vi "Output on.vi"(8 "error in (no error)":errorcluster, 10 "Output On":bool, 11 "E3610x in":refnum<class "E3610x.lvclass">) -> (0 "error out":errorcluster, 3 "E3610x out":refnum<class "E3610x.lvclass">)   [LabVIEW 2020, in "E3610x.lvclass"]
uses:
  E3610x.lvclass
  Instrument.lvclass
  C:/Sandbox/RF Bench/Source Code/WiSpry Test Framework/Instruments/Power Supply/Power Supply.lvclass
  C:/Sandbox/RF Bench/Source Code/WiSpry Test Framework/Instruments/Instrument.lvclass
  C:/Sandbox/RF Bench/Source Code/WiSpry Test Framework/Instruments/Power Supply/Keysight E3610x/E3610x.lvclass
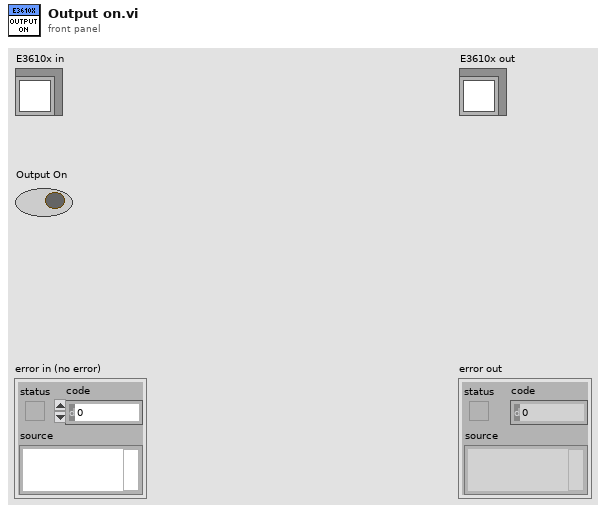
[diagram p1: front panel]
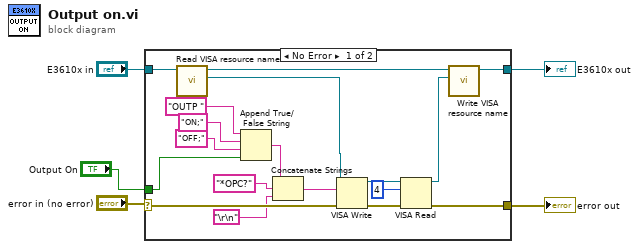
[diagram p0: block diagram]
diagram:
  n1 = case shown="No Error" "error in (no error)" {
    selector: "error in (no error)" -> [w23 w25]
    tunnel: "E3610x in" -> [w22 w24]
    tunnel: "Output On" -> [w20 _]
    tunnel: [w8 w24] -> w2
    tunnel: [w7 w25] -> w1
    frame No Error {
      n2 = call "Read VISA resource name.vi"("Instrument in"=w22) -> ("VISA resource name"=w21:refnum<visa-resource-name>, "Instrument out"=w10:refnum<class "E3610x.lvclass">)  [unwired: 9 in]
      n3 = Append True/False String(1:w20, 2:"OFF;" ("false string"), 3:"ON;" ("true string"), 4:"OUTP " ("string (\"\")")) -> (0:w16:string)
      n4 = Concatenate Strings(w16, "*OPC?" ("string"), "\r\n") -> (w14:string)
      n5 = VISA Write(VISA resource name=w21, write buffer=w14, error in (no error)=w23) -> (VISA resource name out=w12:refnum<visa-resource-name>, error out=w13:errorcluster)  [unwired: 1 out]
      n6 = VISA Read(VISA resource name=w12, byte count=u32 4, error in (no error)=w13) -> (VISA resource name out=w9:refnum<visa-resource-name>, error out=w7:errorcluster)  [unwired: 2 out]
      n7 = call "Write VISA resource name.vi"("VISA resource name"=w9, "Instrument in"=w10) -> ("Instrument out"=w8:refnum<class "E3610x.lvclass">)  [unwired: 9 in]
    }
    frame Error {
    }
  }
  "error out" <- w1
  "E3610x out" <- w2
